vi "NanonisFrametest.vi"(0 "PIN":dbl) -> (4 "POUT":dbl, 6 "FO X":dbl, 8 "FO Z":dbl, 10 "FW":dbl, 15 "FH":dbl)   [LabVIEW 2017]
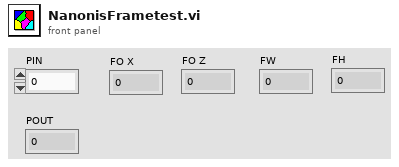
[diagram p1: front panel]
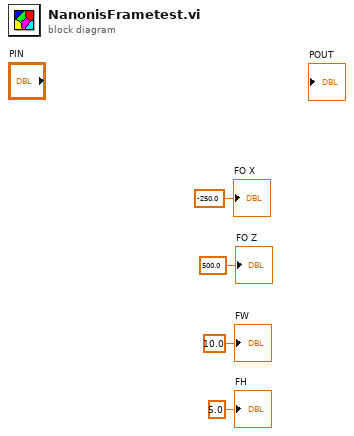
[diagram p0: block diagram]
diagram:
  "FO X" <- -250.0 ("FO X")
  "FO Z" <- 500.0 ("FO Y")
  "FH" <- 5.0 ("FH")
  "FW" <- 10.0 ("FW")
